vi "Add Filter.vi"(10 "Filter":T1 {"End" format="%x"; "Start" format="%x"}, 11 "Filter in":T2(array[cluster]) {"End" format="%x"; "Start" format="%x"}) -> (1 "NewIndex":i32, 2 "Success":bool, 3 "Filter out":T2(array[cluster]) {"End" format="%x"; "Start" format="%x"})   [LabVIEW 2018, in "CAN FD.lvlib"]
uses:
  CAN FD.lvlib
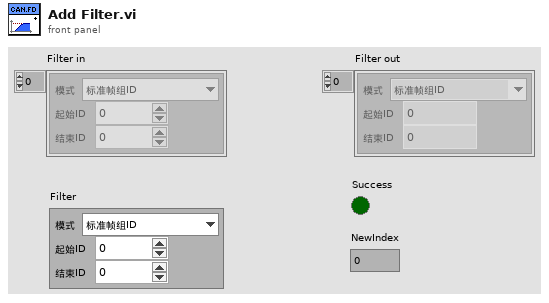
[diagram p1: front panel]
types:
  T1 = cluster{"Mode":enum16{"标准帧组ID", "标准帧明确ID", "扩展帧组ID", "扩展帧明确ID"}, "Start":u32, "End":u32}
  T2 = cluster{"Mode":enum16{"标准帧组ID", "标准帧明确ID", "扩展帧组ID", "扩展帧明确ID"}, "Start":u32, "End":u32}[]
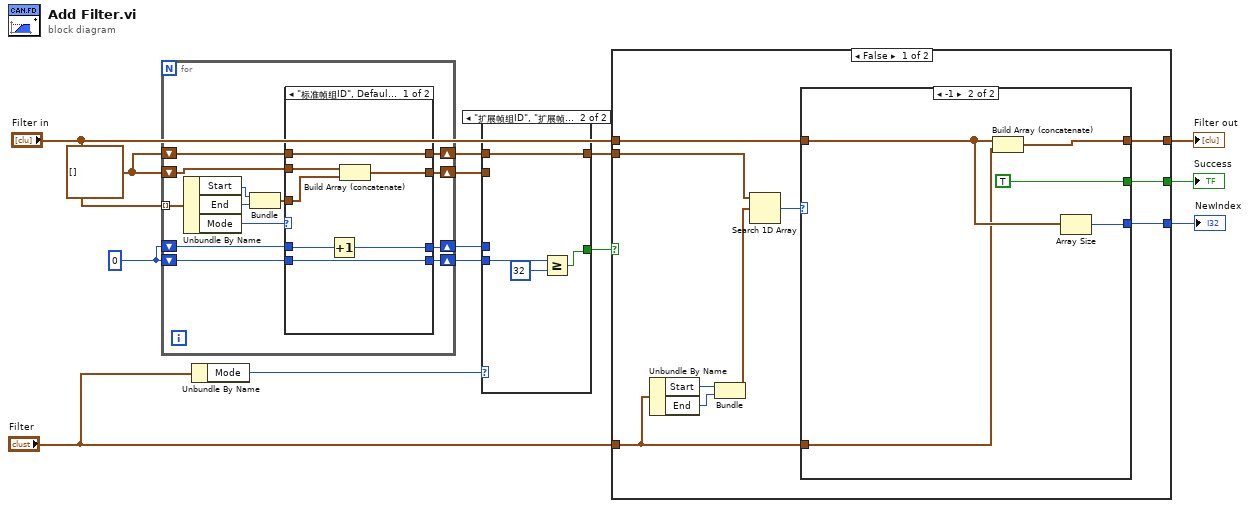
[diagram p0: block diagram]
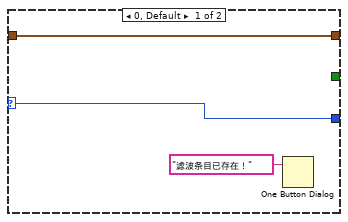
[diagram p2: hidden frame]
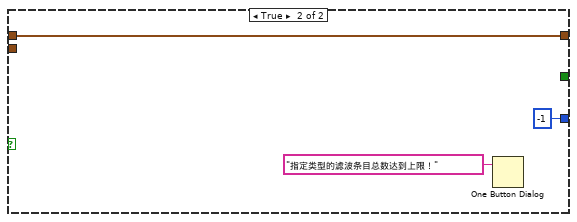
[diagram p3: hidden frame]
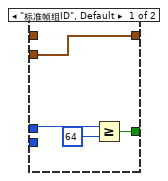
[diagram p4: hidden frame]
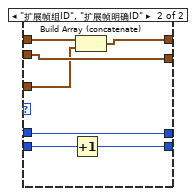
[diagram p5: hidden frame]
diagram:
  w4 = cluster{"Start":u32, "End":u32}[] []
  w14 = 0
  n1 = for {
    tunnel: "Filter in" -> [w27] mode=indexing
    shift-right: [w24] -> w11
    shift-left: w14 -> [w25]
    shift-right: [w22] -> w12
    shift-left: w14 -> [w23]
    shift-right: [w18] -> w1
    shift-left: w4 -> [w17]
    shift-right: [w15] -> w2
    shift-left: w4 -> [w16]
    n2 = Unbundle By Name(w27) -> ("Start"=w20:u32, "End"=w21:u32, "Mode"=w26:enum16{"标准帧组ID", "标准帧明确ID", "扩展帧组ID", "扩展帧明确ID"})
    n3 = Bundle("Start"=w20, "End"=w21) -> (w19:cluster{"Start":u32, "End":u32})  [unwired: 1 in]
    n4 = case shown="\"标准帧组ID\", Default" w26 {
      tunnel: w25 -> [w34 w41]
      tunnel: [w34 w40] -> w24
      tunnel: w23 -> [w33 w39]
      tunnel: [w32 w39] -> w22
      tunnel: w19 -> [w31 w36]
      tunnel: [w30 w38] -> w18
      tunnel: w17 -> [w29 w38]
      tunnel: w16 -> [w28 w37]
      tunnel: [w28 w35] -> w15
      frame "标准帧组ID", Default {
        n5 = Increment(x=w33) -> (x+1=w32:i32)
        n6 = Build Array (concatenate)(w29, w31) -> (w30:cluster{"Start":u32, "End":u32}[])
      }
      frame "扩展帧组ID", "扩展帧明确ID" {
        n7 = Increment(x=w41) -> (x+1=w40:i32)
        n8 = Build Array (concatenate)(w37, w36) -> (w35:cluster{"Start":u32, "End":u32}[])
      }
    }
  }
  n9 = Unbundle By Name("Filter") -> ("Mode"=w13:enum16{"标准帧组ID", "标准帧明确ID", "扩展帧组ID", "扩展帧明确ID"})
  n10 = case shown="\"扩展帧组ID\", \"扩展帧明确ID\"" w13 {
    tunnel: w12 -> [w45 _]
    tunnel: [w43 w47] -> w10
    tunnel: w11 -> [_ w49]
    tunnel: [w42 w46] -> w3
    tunnel: w2 -> [_ w46]
    tunnel: w1 -> [w42 _]
    frame "标准帧组ID", Default {
      n11 = Greater Or Equal?(x=w45, y=64) -> (x >= y?=w43:bool)
    }
    frame "扩展帧组ID", "扩展帧明确ID" {
      n12 = Greater Or Equal?(x=w49, y=32) -> (x >= y?=w47:bool)
    }
  }
  n13 = case shown="False" w10 {
    tunnel: "Filter in" -> [w57 w69]
    tunnel: "Filter" -> [w53 _]
    tunnel: [w59 w69] -> w7
    tunnel: [w58 _] -> w6
    tunnel: [w56 -1 ("index of element")] -> w5
    tunnel: w3 -> [w52 _]
    frame False {
      n14 = Unbundle By Name(w53) -> ("Start"=w55:u32, "End"=w54:u32)
      n15 = Bundle("Start"=w55, "End"=w54) -> (w51:cluster{"Start":u32, "End":u32})  [unwired: 1 in]
      n16 = Search 1D Array(1D array=w52, element=w51) -> (index of element=w50:i32)  [unwired: 1 in]
      n17 = case shown="-1" w50 {
        selector: w50 -> [w60 _]
        tunnel: [w62 w67] -> w59
        tunnel: [_ TRUE] -> w58
        tunnel: w57 -> [w62 w65]
        tunnel: w53 -> [_ w63]
        tunnel: [w60 w64] -> w56
        frame 0, Default {
          n18 = One Button Dialog(message="滤波条目已存在！" ("消息")) -> ()  [unwired: 1 in, 1 out]
        }
        frame -1 {
          n19 = Build Array (concatenate)(w65, w63) -> (w67:T2)
          n20 = Array Size(array=w65) -> (size(s)=w64:i32)
        }
      }
    }
    frame True {
      n21 = One Button Dialog(message="指定类型的滤波条目总数达到上限！" ("消息")) -> ()  [unwired: 1 in, 1 out]
    }
  }
  "Filter out" <- w7
  "Success" <- w6
  "NewIndex" <- w5
